vi "req.vi"() -> ()   [LabVIEW 2014]
uses:
  <vilib>/addons/zeromq/socket_type.ctl
  <userlib>/_OpenG.lib/numeric/numeric.llb/Random Number Within Range - DBL__ogtk.vi
  <vilib>/addons/zeromq/zmq_context.lvclass
  <vilib>/addons/zeromq/zeromq.lvlib
  <vilib>/addons/zeromq/zmq_socket.lvclass
panel:
  in  "iter_num":i32=2
  out "concatenated string":string
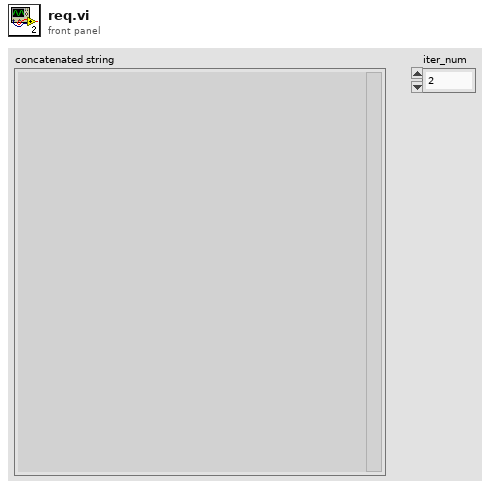
[diagram p1: front panel]
types:
  T1 = typedef "zeromq.lvlib/socket_type.ctl" = enum8{"ZMQ_PAIR", "ZMQ_PUB", "ZMQ_SUB", "ZMQ_REQ", "ZMQ_REP", "ZMQ_DEALER", "ZMQ_ROUTER", "ZMQ_PULL", "ZMQ_PUSH", "ZMQ_XPUB", "ZMQ_XSUB"}
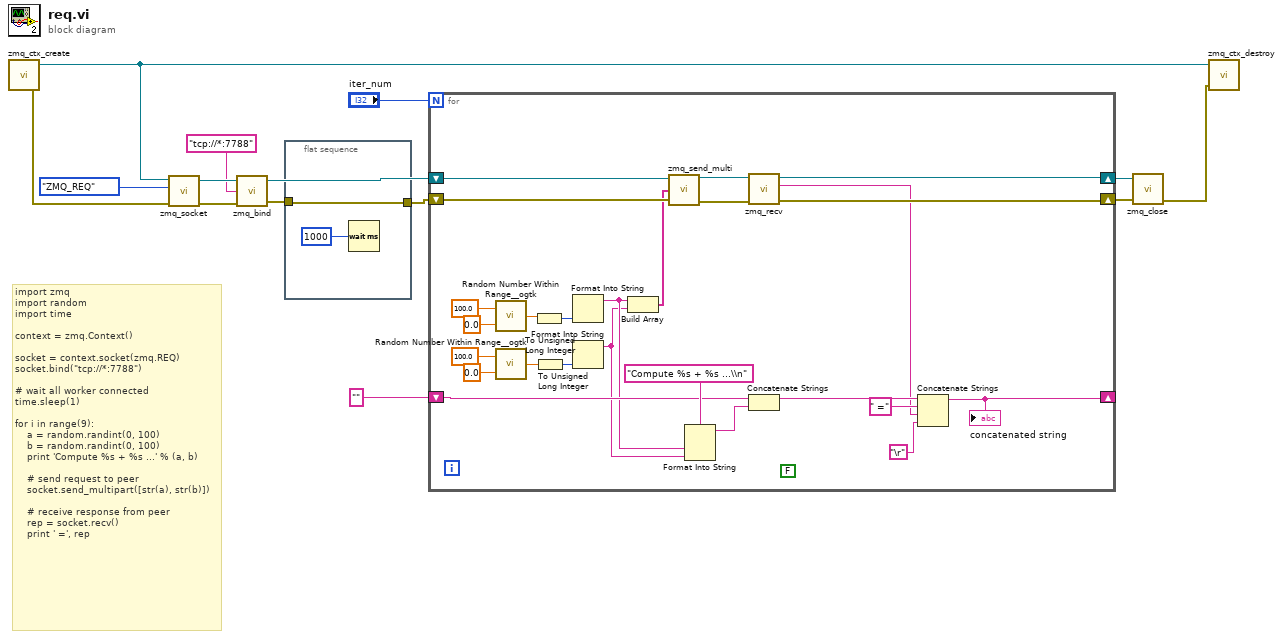
[diagram p0: block diagram]
diagram:
  # "import zmq\nimport random\nimport time\n\ncontext = zmq.Context()\n\nsocket = context.socket(zmq.REQ)\nsocket.bind(\"tcp://*:7788\")\n\n# wait all worker connected\ntime.sleep(1)\n\nfor i in range(9):\n    a = random.randint(0, 100)\n    b = random.randint(0, 100)\n    print 'Compute %s + %s ...' % (a, b)\n\n    # send request to peer\n    socket.send_multipart([str(a), str(b)])\n\n    # receive response from peer\n    rep = socket.recv()\n    print ' =', rep"
  n1 = call <vilib>:"zmq_ctx_create.vi"() -> ("error out"=w13:errorcluster, "context out"=w12:refnum<class "zmq_context.lvclass">)  [unwired: 4 in]
  n2 = call <vilib>:"zmq_socket.vi"("error in"=w13, "socket type"=socket_type."ZMQ_REQ", "context in"=w12) -> ("error out"=w10:errorcluster, "socket out"=w11:refnum<class "zmq_socket.lvclass">)  [unwired: 2 in, 1 out]
  n3 = call <vilib>:"zmq_bind.vi"("error in"=w10, "endpoint"="tcp://*:7788", "socket in"=w11) -> ("error out"=w3:errorcluster, "socket out"=w7:refnum<class "zmq_socket.lvclass">)  [unwired: 1 in]
  n4 = flat-sequence {
    tunnel: [w15] -> w4
    tunnel: w3 -> [w15]
    frame #0 {
      n5 = Wait (ms)(milliseconds to wait=u32 1000) -> ()  [unwired: 1 out]
    }
  }
  n6 = for {
    N: "iter_num" -> [_]
    shift-right: [w38] -> w6
    shift-left: w7 -> [w41]
    shift-right: [w37] -> w5
    shift-left: w4 -> [w36]
    shift-right: [w20] -> _
    shift-left: "" -> [w24]
    (unwired) FALSE
    n7 = call-poly <userlib>:"Random Number Within Range__ogtk.vi"("High"=100.0, "Low"=0.0) -> ("Random Number"=w31:dbl)  [unwired: 3 in]
    n8 = call-poly <userlib>:"Random Number Within Range__ogtk.vi"("High"=100.0, "Low"=0.0) -> ("Random Number"=w30:dbl)  [unwired: 3 in]
    n9 = To Unsigned Long Integer(number=w31) -> (unsigned 32bit integer=w29:u32)
    n10 = To Unsigned Long Integer(number=w30) -> (unsigned 32bit integer=w28:u32)
    n11 = Format Into String(w29) -> (resulting string=w23:string)  [unwired: 3 in, 1 out]
    n12 = Format Into String(w28) -> (resulting string=w22:string)  [unwired: 3 in, 1 out]
    n13 = Build Array(w23, w22) -> (w27:string[])
    n14 = call <vilib>:"zmq_send_multi.vi"("error in"=w36, "parts"=w27, "socket in"=w41) -> ("error out"=w40:errorcluster, "socket out"=w39:refnum<class "zmq_socket.lvclass">)  [unwired: 1 in]
    n15 = Format Into String(format string="Compute %s + %s ...\\n", w23, w22) -> (resulting string=w26:string)  [unwired: 2 in, 1 out]
    n16 = call <vilib>:"zmq_recv.vi"("error in"=w40, "socket in"=w39) -> ("error out"=w37:errorcluster, "data"=w18:string, "socket out"=w38:refnum<class "zmq_socket.lvclass">)  [unwired: 3 in, 2 out]
    n17 = Concatenate Strings(w24, w26) -> (w21:string)
    n18 = Concatenate Strings(w21, " =" ("string"), w18, "\r") -> (w20:string)
    "concatenated string" <- w20
  }
  n19 = call <vilib>:"zmq_close.vi"("error in"=w5, "socket"=w6) -> ("error out"=w8:errorcluster)  [unwired: 3 in]
  n20 = call <vilib>:"zmq_ctx_destroy.vi"("error in"=w8, "context in"=w12) -> ()  [unwired: 3 in, 1 out]
